vi "AFEBasicTest.vi"() -> ()   [LabVIEW 2017]
uses:
  <vilib>/rvi/interface/nirviOpenFPGA/nirviOpenFPGA.xnode
  <vilib>/rvi/interface/nirviCloseFPGA/nirviCloseFPGA.xnode
  <vilib>/rvi/interface/nirviMethod/nirviMethod.xnode
  <vilib>/NI/PowerElectronicsControl/ScaleAndLimit/Interface/ScaleAndLimitInterface.lvlib
  <vilib>/NI/PowerElectronicsControl/ScaleAndLimit/Interface/Configuration.ctl
  <vilib>/rvi/interface/nirviReadWriteControl/nirviReadWriteControl.xnode
  <instrlib>/_niInstr/FIFO Register Bus/v1/Host/niInstr FIFO Register Bus v1 Host.lvclass
  <instrlib>/_niInstr/Instruction Framework/v1/Host/Subsystem Map/niInstr Subsystem Map v1 Host.lvclass
  <vilib>/FPGAPlugInAG/Dynamic/niLvFpga_Run_Dynamic.vi
  <vilib>/NI/PowerElectronicsControl/WaveformAcq/RT/WaveformTask.lvclass
  <vilib>/Utility/error.llb/Error Cluster From Error Code.vi
  <vilib>/rvi/interface/Simulation/niFpgaSimulationCallBeginRW.vi
  <vilib>/rvi/errors/niLvFpgaAdjustHostInterfaceError.vi
  <vilib>/NI/PowerElectronicsControl/SVPWM/SVPWMInterface/SVPWMInterface.lvlib
  <vilib>/NI/PowerElectronicsControl/WaveformAcq/RT/ReadWaveform.vi
  C:/Program Files (x86)/National Instruments/LabVIEW 2017/instr.lib/_niInstr/Instruction Framework/v1/Host/Instruction Target/niInstr Instruction Target v1 Host.lvclass
  NiFpgaLv.dll
  <vilib>/FPGAPlugInAG/Dynamic/niLvFpga_Close_Dynamic.vi
  FPGA Bitfiles/AFE_FPGATarget_CoreTestHarness_iG140jQplF0.lvbitx
  tests/CoreTestHarness.vi
  <vilib>/FPGAPlugInAG/sbRIO-9607/niLvFpga_Open_sbRIO-9607.vi
  <vilib>/rvi/interface/common/dynamic/niFpgaDynamicAddResources.vi
panel:
  in  "Pause":bool
  in  "UpdateRate":dbl
  in  "Tabs":T1(tab)
  out "General":waveform(sgl)[](graph)
  out "PLL Tuning":waveform(sgl)[](graph)
  out "Icmd to Vcmd":waveform(sgl)[](graph)
  out "VDCLink to Icmd":waveform(sgl)[](graph)
  in  "UpdateSettings":bool
  in  "AFE_Setpoints":cluster{"VDCLink":sgl, "DirectedIdSetpt":sgl}
  in  "AFE_Gains":T2
  in  "AFE_ManualControl":T3
  in  "AFE_ControlSignals":cluster{"resetPLL":bool, "resetControl":bool}
  out "actualAFErate":i16
  in  "enableIGBTs":bool
  out "Limits":string
  out "SimultaneousAILoopRate":u32
  in  "clearLimits":bool
  in  "stop":bool
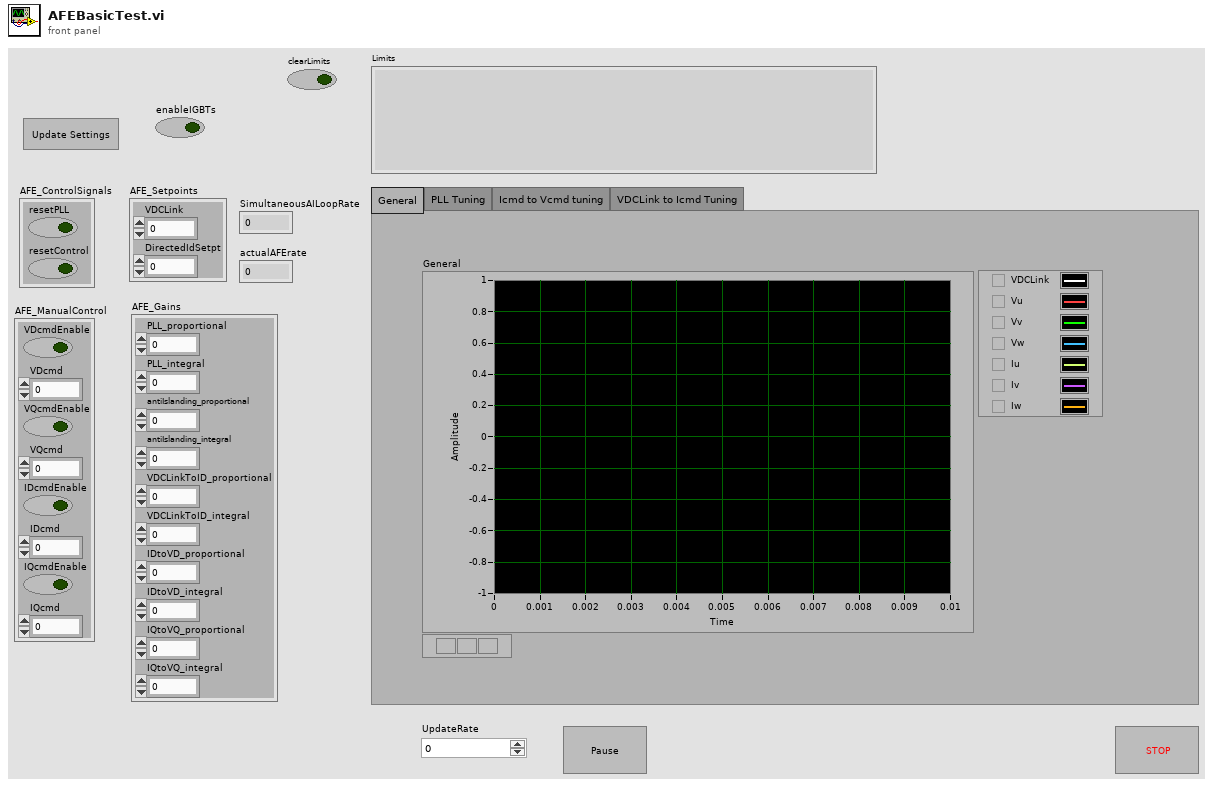
[diagram p1: front panel]
types:
  T1 = enum32{"General", "PLL Tuning", "Icmd to Vcmd tuning", "VDCLink to Icmd Tuning"}
  T2 = cluster{"PLL_proportional":sgl, "PLL_integral":sgl, "antiIslanding_proportional":sgl, "antiIslanding_integral":sgl, "VDCLinkToID_proportional":sgl, "VDCLinkToID_integral":sgl, "IDtoVD_proportional":sgl, "IDtoVD_integral":sgl, "IQtoVQ_proportional":sgl, "IQtoVQ_integral":sgl}
  T3 = cluster{"VDcmdEnable":bool, "VDcmd":sgl, "VQcmdEnable":bool, "VQcmd":sgl, "IDcmdEnable":bool, "IDcmd":sgl, "IQcmdEnable":bool, "IQcmd":sgl}
  T4 = cluster{"GridExpectedFreq":sgl, "dT":sgl, "DirectIdCntrl":bool, "AntiIslanding":bool}
  T5 = cluster{"PLL_PIRad_high":sgl, "PLL_PiRad_low":sgl, "IQcmd_high":sgl, "IQcmd_low":sgl, "IDcmd_high":sgl, "IDcmd_low":sgl, "VDcmd_high":sgl, "VDcmd_low":sgl, "VQmcd_high":sgl, "VQcmd_low":sgl}
  T6 = typedef "ScaleAndLimitInterface.lvlib/Configuration.ctl" = cluster{"Name":string, "M":dbl, "B":i16, "HighLimit":dbl, "LowLimit":dbl, "LimitsEnabled":bool}
  T7 = typedef "SVPWMInterface.lvlib/Configuration.ctl" = cluster{"Deadtime":u8, "Period":u32}
  T8 = typedef "ScaleAndLimitInterface.lvlib/Interface.ctl" = cluster{"instruction target":refnum<class "niInstr Instruction Target v1 Host.lvclass">, "ScalingAndLimitsContext":refnum<class "niInstr Instruction Framework Context v1 Host.lvclass">, "Configuration":T6[]}
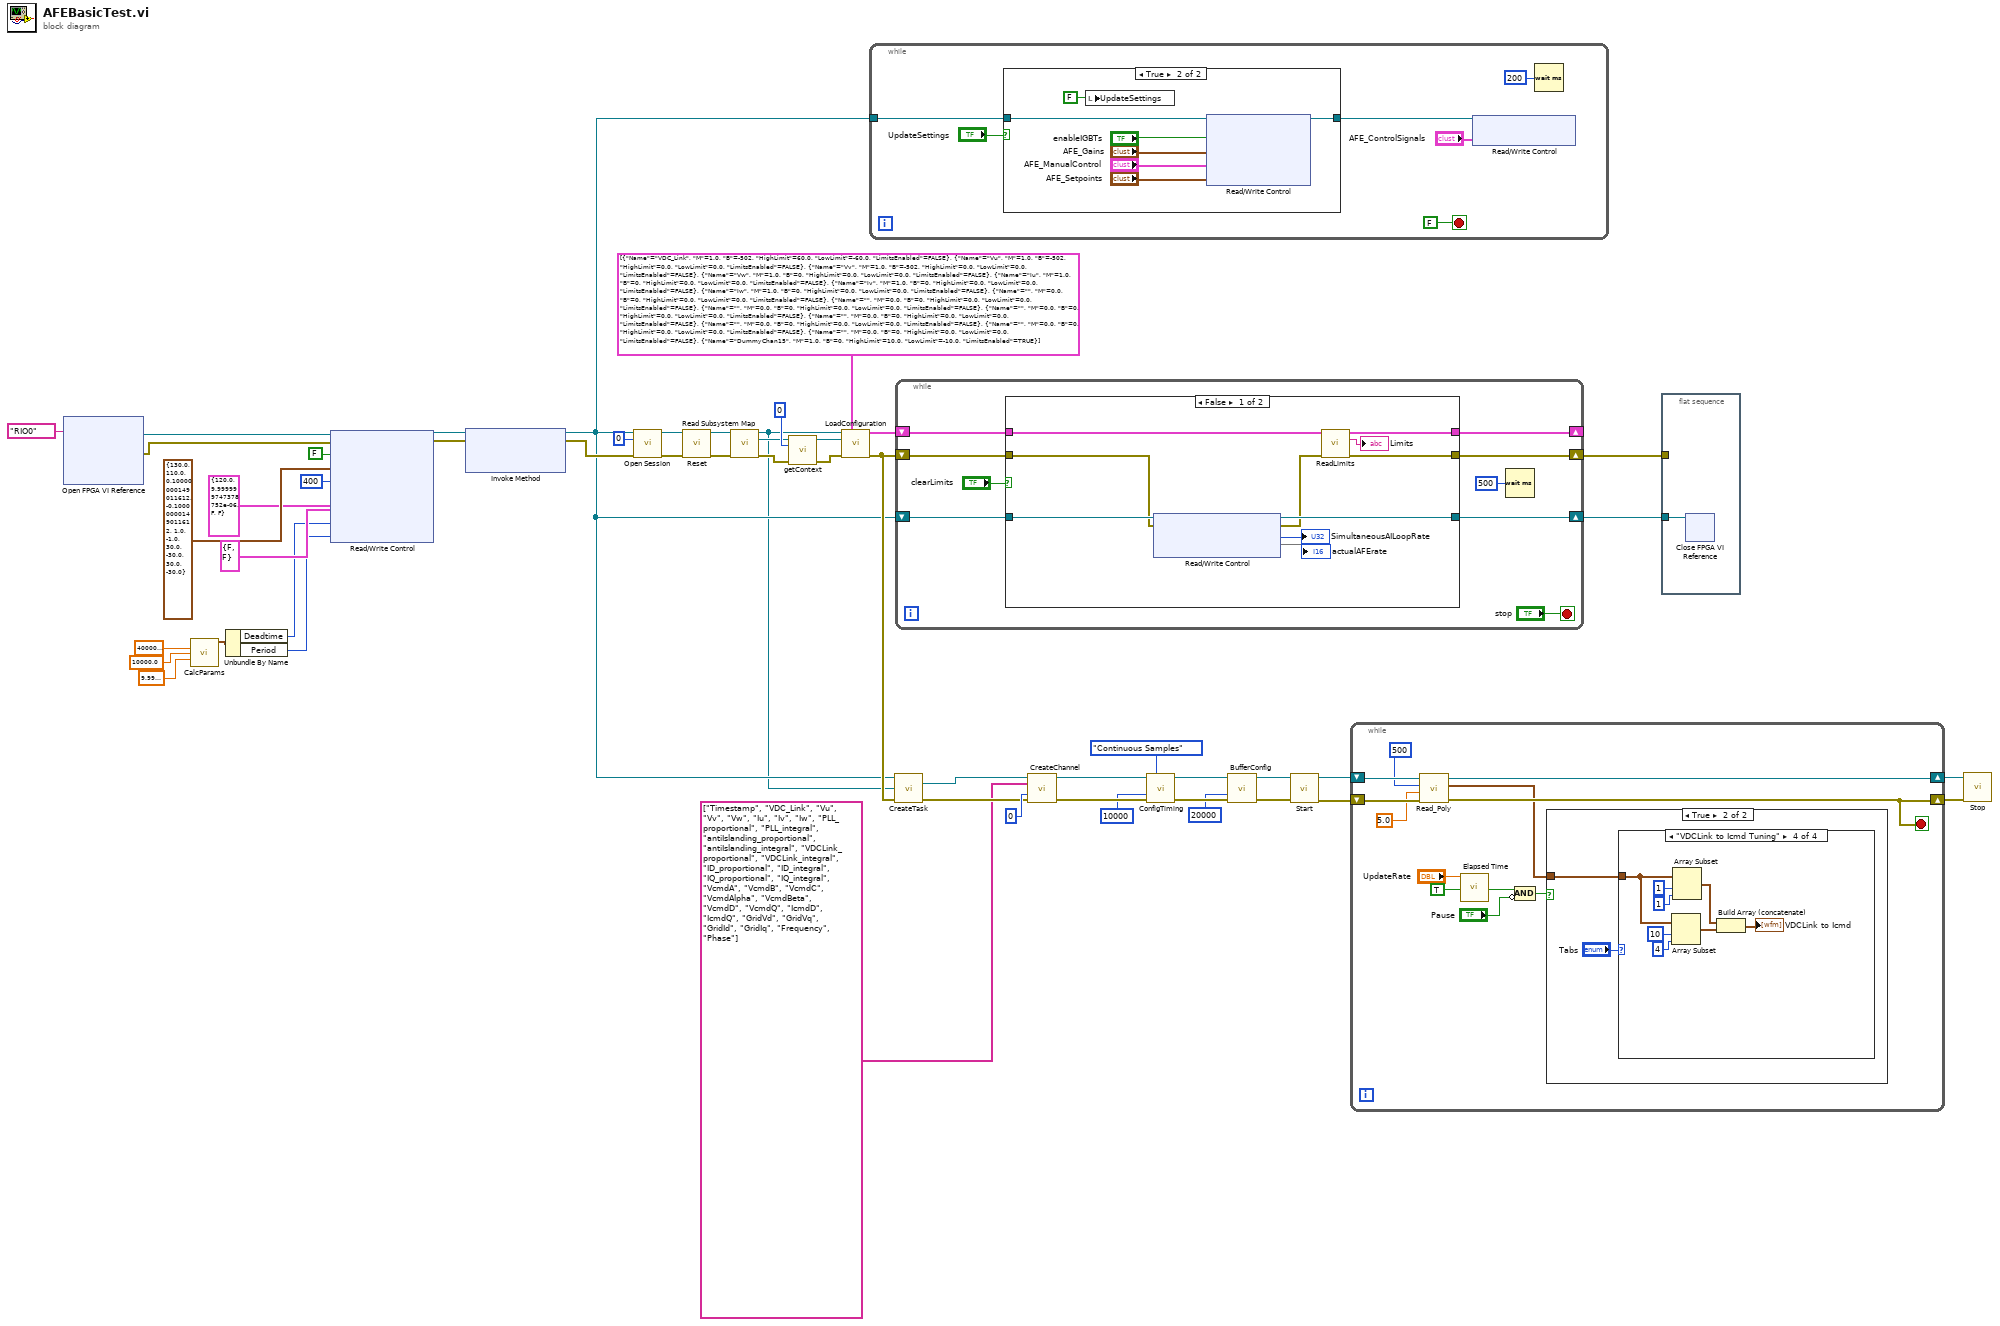
[diagram p0: block diagram]
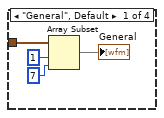
[diagram p4: hidden frame]
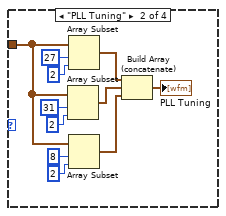
[diagram p5: hidden frame]
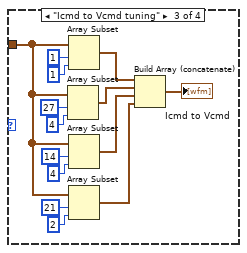
[diagram p6: hidden frame]
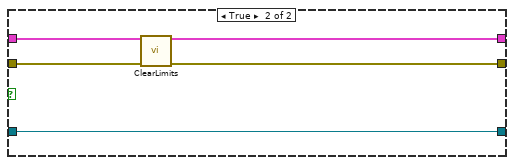
[diagram p7: hidden frame]
diagram:
  n1 = xnode "Open FPGA VI Reference"("resource name"=tag "RIO0") -> ("FPGA VI Reference Out"=w19:refnum<k20>, "error out"=w18:errorcluster)  [unwired: 1 in]
  n2 = call <vilib>:"CalcParams.vi"("ClkRate"=sgl 40000000.0, "fc"=sgl 10000.0, "deadtime"=sgl 1e-06) -> ("Configuration"=w7:T7)  [unwired: 12 in]
  n3 = Unbundle By Name(w7) -> ("Deadtime"=w6:u8, "Period"=w5:u32)
  n4 = xnode "Read/Write Control"("FPGA VI Reference In"=w19, "error in"=w18, "enableIGBTs"=FALSE, "AFE_Range"=T5 {"PLL_PIRad_high"=130.0, "PLL_PiRad_low"=110.0, "IQcmd_high"=0.1, "IQcmd_low"=-0.1, "IDcmd_high"=1.0, "IDcmd_low"=-1.0, "VDcmd_high"=30.0, "VDcmd_low"=-30.0, "VQmcd_high"=30.0, "VQcmd_low"=-30.0}, "AFE_rate"=i16 400, "AFE_Params"=T4 {"GridExpectedFreq"=120.0, "dT"=1e-05, "DirectIdCntrl"=FALSE, "AntiIslanding"=FALSE}, "AFE_ControlSignals"=cluster{"resetPLL":bool, "resetControl":bool} {"resetPLL"=FALSE, "resetControl"=FALSE}, "Deadtime"=w6, "Period"=w5) -> ("FPGA VI Reference Out"=w17:refnum<k20>, "error out"=w16:errorcluster)
  n5 = xnode "Invoke Method"("FPGA VI Reference In"=w17, "error in"=w16) -> ("FPGA VI Reference Out"=w4:refnum<k20>, "error out"=w41:errorcluster)  [unwired: 1 in]
  n6 = call <instrlib>:"Open Session.vi"("fpga ref"=w4, "bus instance"=u32 0, "error in"=w41) -> ("session out"=w45:refnum<class "niInstr FIFO Register Bus v1 Host.lvclass">, "error out"=w46:errorcluster)  [unwired: 11 in]
  n7 = call-dynamic "Reset.vi"("session in"=w45, "error in"=w46) -> ("session out"=w22:refnum<class "niInstr FIFO Register Bus v1 Host.lvclass">, "error out"=w44:errorcluster)  [unwired: 12 in]
  n8 = call <instrlib>:"Read Subsystem Map.vi"("instruction target in"=w22, "error in"=w44) -> ("instruction target out"=w1:refnum<class "niInstr FIFO Register Bus v1 Host.lvclass">, "subsystem map"=w3:refnum<class "niInstr Subsystem Map v1 Host.lvclass">, "error out"=w43:errorcluster)  [unwired: 11 in]
  n9 = call <vilib>:"getContext.vi"("subsystemMap"=w3, "instance"=u8 0, "error in"=w43) -> ("ScalingAndLimitsContext"=w2:refnum<class "niInstr Instruction Framework Context v1 Host.lvclass">, "error out"=w50:errorcluster)  [unwired: 11 in]
  n10 = call <vilib>:"LoadConfiguration.vi"("instruction target in"=w1, "Configuration"=T6[] [{"Name"="VDC_Link", "M"=1.0, "B"=-502, "HighLimit"=60.0, "LowLimit"=-60.0, "LimitsEnabled"=FALSE}, {"Name"="Vu", "M"=1.0, "B"=-502, "HighLimit"=0.0, "LowLimit"=0.0, "LimitsEnabled"=FALSE}, {"Name"="Vv", "M"=1.0, "B"=-502, "HighLimit"=0.0, "LowLimit"=0.0, "LimitsEnabled"=FALSE}, {"Name"="Vw", "M"=1.0, "B"=0, "HighLimit"=0.0, "LowLimit"=0.0, "LimitsEnabled"=FALSE}, {"Name"="Iu", "M"=1.0, "B"=0, "HighLimit"=0.0, "LowLimit"=0.0, "LimitsEnabled"=FALSE}, {"Name"="Iv", "M"=1.0, "B"=0, "HighLimit"=0.0, "LowLimit"=0.0, "LimitsEnabled"=FALSE}, {"Name"="Iw", "M"=1.0, "B"=0, "HighLimit"=0.0, "LowLimit"=0.0, "LimitsEnabled"=FALSE}, {"Name"="", "M"=0.0, "B"=0, "HighLimit"=0.0, "LowLimit"=0.0, "LimitsEnabled"=FALSE}, {"Name"="", "M"=0.0, "B"=0, "HighLimit"=0.0, "LowLimit"=0.0, "LimitsEnabled"=FALSE}, {"Name"="", "M"=0.0, "B"=0, "HighLimit"=0.0, "LowLimit"=0.0, "LimitsEnabled"=FALSE}, {"Name"="", "M"=0.0, "B"=0, "HighLimit"=0.0, "LowLimit"=0.0, "LimitsEnabled"=FALSE}, {"Name"="", "M"=0.0, "B"=0, "HighLimit"=0.0, "LowLimit"=0.0, "LimitsEnabled"=FALSE}, {"Name"="", "M"=0.0, "B"=0, "HighLimit"=0.0, "LowLimit"=0.0, "LimitsEnabled"=FALSE}, {"Name"="", "M"=0.0, "B"=0, "HighLimit"=0.0, "LowLimit"=0.0, "LimitsEnabled"=FALSE}, {"Name"="", "M"=0.0, "B"=0, "HighLimit"=0.0, "LowLimit"=0.0, "LimitsEnabled"=FALSE}, {"Name"="DummyChan15", "M"=1.0, "B"=0, "HighLimit"=10.0, "LowLimit"=-10.0, "LimitsEnabled"=TRUE}], "ScalingAndLimitsContext"=w2, "error in (no error)"=w50) -> ("Interface"=w47:T8, "error out"=w21:errorcluster)  [unwired: 10 in]
  n11 = while {
    tunnel: w4 -> [w57]
    stop <- FALSE stop-if-true
    n12 = case shown="True" "UpdateSettings" {
      tunnel: w57 -> [w58 w65]
      tunnel: [w58 w59] -> w53
      frame False {
      }
      frame True {
        n13 = local write "UpdateSettings"(FALSE ("UpdateSettings")) -> ()
        n14 = xnode "Read/Write Control"("FPGA VI Reference In"=w65, "enableIGBTs"="enableIGBTs", "AFE_Gains"="AFE_Gains", "AFE_ManualControl"="AFE_ManualControl", "AFE_Setpoints"="AFE_Setpoints") -> ("FPGA VI Reference Out"=w59:refnum<k20>)  [unwired: 1 in, 1 out]
      }
    }
    n15 = xnode "Read/Write Control"("FPGA VI Reference In"=w53, "AFE_ControlSignals"="AFE_ControlSignals") -> ()  [unwired: 1 in, 2 out]
    n16 = Wait (ms)(milliseconds to wait=u32 200) -> ()  [unwired: 1 out]
  }
  n17 = call <vilib>:"CreateTask.vi"("FPGA Ref in"=w4, "session in"=w1, "error in"=w21) -> ("Task out"=w26:refnum<class "WaveformTask.lvclass">, "error out"=w25:errorcluster)  [unwired: 9 in, 2 out]
  n18 = while {
    shift-right: [w67] -> _
    shift-left: w47 -> [w74]
    shift-right: [w66] -> w39
    shift-left: w21 -> [w73]
    shift-right: [w68] -> w40
    shift-left: w4 -> [w69]
    stop <- "stop" stop-if-true
    n19 = case shown="False" "clearLimits" {
      tunnel: w74 -> [w81 w89]
      tunnel: w73 -> [w83 w88]
      tunnel: [w80 w87] -> w67
      tunnel: [w79 w86] -> w66
      tunnel: w69 -> [w84 w85]
      tunnel: [w82 w85] -> w68
      frame False {
        n20 = xnode "Read/Write Control"("FPGA VI Reference In"=w84, "error in"=w83) -> ("FPGA VI Reference Out"=w82:refnum<k20>, "error out"=w77:errorcluster, "SimultaneousAILoopRate"=→"SimultaneousAILoopRate":u32, "actualAFErate"=→"actualAFErate")
        n21 = call <vilib>:"ReadLimits.vi"("Interface in"=w81, "error in (no error)"=w77) -> ("Interface out"=w80:T8, "Limits"=→"Limits":string, "error out"=w79:errorcluster)  [unwired: 11 in]
      }
      frame True {
        n22 = call <vilib>:"ClearLimits.vi"("Interface in"=w89, "error in (no error)"=w88) -> ("Interface out"=w87:T8, "error out"=w86:errorcluster)  [unwired: 12 in]
      }
    }
    n23 = Wait (ms)(milliseconds to wait=u32 500) -> ()  [unwired: 1 out]
  }
  n24 = call <vilib>:"CreateChannel.vi"("task in"=w26, "Chan Name Array"=string[] ["Timestamp", "VDC_Link", "Vu", "Vv", "Vw", "Iu", "Iv", "Iw", "PLL_proportional", "PLL_integral", "antiIslanding_proportional", "antiIslanding_integral", "VDCLink_proportional", "VDCLink_integral", "ID_proportional", "ID_integral", "IQ_proportional", "IQ_integral", "VcmdA", "VcmdB", "VcmdC", "VcmdAlpha", "VcmdBeta", "VcmdD", "VcmdQ", "IcmdD", "IcmdQ", "GridVd", "GridVq", "GridId", "GridIq", "Frequency", "Phase"], "instance"=u8 0, "error in"=w25) -> ("Task out"=w27:refnum<class "WaveformTask.lvclass">, "error out"=w37:errorcluster)  [unwired: 10 in]
  n25 = call <vilib>:"ConfigTiming.vi"("Task in"=w27, "Sample Mode"=enum16{"Finite Samples", "Continuous Samples"}."Continuous Samples", "Sample Rate"=u32 10000, "error in (no error)"=w37) -> ("Task out"=w34:refnum<class "WaveformTask.lvclass">, "error out"=w33:errorcluster)  [unwired: 9 in, 1 out]
  n26 = call <vilib>:"BufferConfig.vi"("WaveformTask in"=w34, "Buffer Size [Samps per Chan]"=20000, "error in (no error)"=w33) -> ("WaveformTask out"=w31:refnum<class "WaveformTask.lvclass">, "error out"=w30:errorcluster)  [unwired: 10 in, 1 out]
  n27 = call <vilib>:"Start.vi"("WaveformTask in"=w31, "error in (no error)"=w30) -> ("WaveformTask out"=w29:refnum<class "WaveformTask.lvclass">, "error out"=w28:errorcluster)  [unwired: 12 in]
  n28 = while {
    shift-right: [w96] -> w23
    shift-left: w28 -> [w100]
    shift-right: [w97] -> w24
    shift-left: w29 -> [w101]
    stop <- w96 stop-if-true
    n29 = call-poly <vilib>:"Read_Poly.vi"("error in"=w100, "Timeout (s)"=5.0, "Samps Read per Chan"=500, "Task in"=w101) -> ("error out"=w96:errorcluster, "Waveforms"=w90:waveform(sgl)[], "Task out"=w97:refnum<class "WaveformTask.lvclass">)  [unwired: 4 in, 1 out]
    n30 = call "Elapsed Time"("Time Target (s)"="UpdateRate", "Auto Reset"=TRUE) -> ("Time has Elapsed"=w94:bool)  [unwired: 10 in, 7 out]
    n31 = Compound Arithmetic op=AND(w94, invert "Pause") -> (w91:bool)
    n32 = case shown="True" w91 {
      tunnel: w90 -> [_ w102]
      frame False {
      }
      frame True {
        n33 = case shown="\"VDCLink to Icmd Tuning\"" "Tabs" {
          tunnel: w102 -> [w105 w112 w121 w134]
          frame "General", Default {
            n34 = Array Subset(array=w105, index=1, length=7) -> (→"General":waveform(sgl)[])
          }
          frame "PLL Tuning" {
            n35 = Array Subset(array=w112, index=31, length=2) -> (w110:waveform(sgl)[])
            n36 = Array Subset(array=w112, index=27, length=2) -> (w111:waveform(sgl)[])
            n37 = Array Subset(array=w112, index=8, length=2) -> (w109:waveform(sgl)[])
            n38 = Build Array (concatenate)(w111, w110, w109) -> (→"PLL Tuning":waveform(sgl)[])
          }
          frame "Icmd to Vcmd tuning" {
            n39 = Array Subset(array=w121, index=27, length=4) -> (w125:waveform(sgl)[])
            n40 = Array Subset(array=w121, index=1, length=1) -> (w126:waveform(sgl)[])
            n41 = Array Subset(array=w121, index=14, length=4) -> (w124:waveform(sgl)[])
            n42 = Array Subset(array=w121, index=21, length=2) -> (w120:waveform(sgl)[])
            n43 = Build Array (concatenate)(w126, w125, w124, w120) -> (→"Icmd to Vcmd":waveform(sgl)[])
          }
          frame "VDCLink to Icmd Tuning" {
            n44 = Array Subset(array=w134, index=10, length=4) -> (w135:waveform(sgl)[])
            n45 = Array Subset(array=w134, index=1, length=1) -> (w136:waveform(sgl)[])
            n46 = Build Array (concatenate)(w136, w135) -> (→"VDCLink to Icmd":waveform(sgl)[])
          }
        }
      }
    }
  }
  n47 = flat-sequence {
    tunnel: w40 -> [w141]
    tunnel: w39 -> [_]
    frame #0 {
      n48 = xnode "Close FPGA VI Reference"("FPGA VI Reference In"=w141) -> ()  [unwired: 1 in, 1 out]
    }
  }
  n49 = call <vilib>:"Stop.vi"("error in"=w23, "WaveformTask in"=w24) -> ()  [unwired: 8 in, 2 out]
